vi "Agilent VNA Set Trigger Mode.vi"(6 "Channel":i8=1 min=1 max=99 step=1, 7 "Agilent VNA":T1, 8 "error in (no error)":errorcluster, 10 "Trigger Mode":T2, 11 "VISA Resource Name":refnum<visa-resource-name>) -> (0 "error out":errorcluster, 3 "dup VISA Resource Name":refnum<visa-resource-name>)   [LabVIEW 2011]
doc: "This VI for the HP8753B Network Analyzers reads the stimulus values. Except when performing log sweeps and freq list sweeps, this VI uses the start and stop values and the number of points to calcuate the stimulus values."
uses:
  TypeDefs/Agilent VNA Trigger Mode.ctl
  TypeDefs/Agilent VNA Instrument Info.ctl
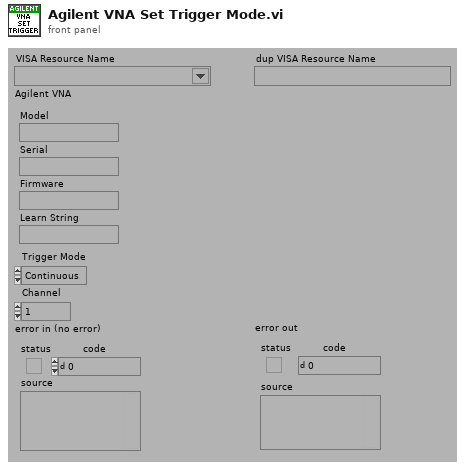
[diagram p1: front panel]
types:
  T1 = typedef "Agilent VNA Instrument Info.ctl" = cluster{"Model":string, "Serial":string, "Firmware":string, "Learn String":string}
  T2 = typedef "Agilent VNA Trigger Mode.ctl" = enum16{"Continuous", "Hold", "Single"}
  T3 = typedef "Agilent VNA Model.ctl" = enum16{"Not Supported", "8510X", "8719X", "8720X", "8722X", "8753X", "ENA", "PNA", "Field Fox"}
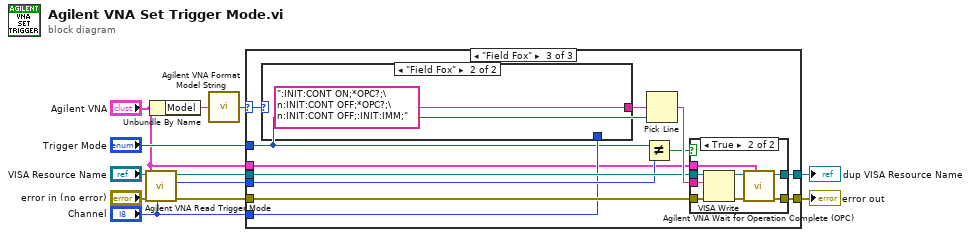
[diagram p0: block diagram]
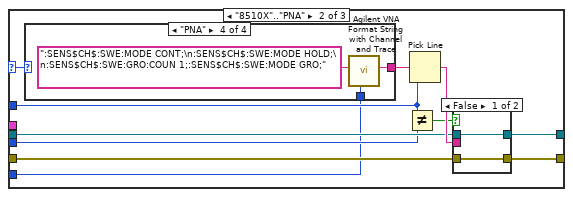
[diagram p3: hidden frame]
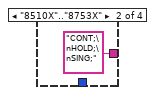
[diagram p5: hidden frame]
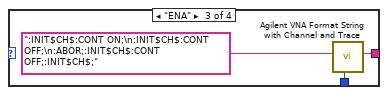
[diagram p6: hidden frame]
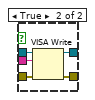
[diagram p7: hidden frame]
diagram:
  n1 = call "Agilent VNA Read Trigger Mode.vi"("Channel"="Channel", "Agilent VNA"="Agilent VNA", "error in (no error)"="error in (no error)", "VISA Resource Name"="VISA Resource Name") -> ("error out"=w7:errorcluster, "Trigger Mode"=w5:T2, "dup VISA Resource Name"=w6:refnum<visa-resource-name>)  [unwired: 5 out]
  n2 = Unbundle By Name("Agilent VNA") -> ("Model"=w3:string)
  n3 = call "Agilent VNA Format Model String.vi"("Model"=w3) -> ("Model"=w2:T3)
  n4 = case shown="\"Field Fox\"" w2 {
    selector: w2 -> [_ w15 w42]
    tunnel: [w13 w25 w51] -> w12
    tunnel: [w14 w24 w50] -> w11
    tunnel: "Trigger Mode" -> [_ w23 w40]
    tunnel: w7 -> [w14 w19 w46]
    tunnel: w6 -> [w13 w18 w45]
    tunnel: w5 -> [_ w17 w44]
    tunnel: "Channel" -> [_ w16 w43]
    tunnel: "Agilent VNA" -> [_ _ w41]
    frame "Not Supported" {
    }
    frame "8510X".."PNA" {
      n5 = case shown="\"PNA\"" w15 {
        tunnel: [_ "CONT;\nHOLD;\nSING;" w28 w31] -> w21
        tunnel: w16 -> [_ _ w27 w30]
        frame "Not Supported", "Field Fox" {
        }
        frame "8510X".."8753X" {
        }
        frame "ENA" {
          n6 = call "Agilent VNA Format String with Channel and Trace.vi"("Channel"=w27, "String"=":INIT$CH$:CONT ON;\n:INIT$CH$:CONT OFF;\n:ABOR;:INIT$CH$:CONT OFF;:INIT$CH$;") -> ("String Out"=w28:string)  [unwired: 1 in, 6 out]
        }
        frame "PNA" {
          n7 = call "Agilent VNA Format String with Channel and Trace.vi"("Channel"=w30, "String"=":SENS$CH$:SWE:MODE CONT;\n:SENS$CH$:SWE:MODE HOLD;\n:SENS$CH$:SWE:GRO:COUN 1;:SENS$CH$:SWE:MODE GRO;") -> ("String Out"=w31:string)  [unwired: 1 in, 6 out]
        }
      }
      n8 = Not Equal?(x=w23, y=w17) -> (x != y?=w20:bool)
      n9 = Pick Line(multi-line string=w21, line index=w23) -> (output string=w22:string)  [unwired: 1 out]
      n10 = case shown="False" w20 {
        tunnel: w19 -> [w33 w39]
        tunnel: w18 -> [w34 w38]
        tunnel: w22 -> [_ w37]
        tunnel: [w34 w36] -> w25
        tunnel: [w33 w35] -> w24
        frame False {
        }
        frame True {
          n11 = VISA Write(VISA resource name=w38, write buffer=w37, error in (no error)=w39) -> (VISA resource name out=w36:refnum<visa-resource-name>, error out=w35:errorcluster)  [unwired: 1 out]
        }
      }
    }
    frame "Field Fox" {
      n12 = case shown="\"Field Fox\"" w42 {
        tunnel: [_ ":INIT:CONT ON;*OPC?;\n:INIT:CONT OFF;*OPC?;\n:INIT:CONT OFF;:INIT:IMM;"] -> w48
        tunnel: w43 -> [_ _]
        frame "Not Supported".."PNA" {
        }
        frame "Field Fox" {
        }
      }
      n13 = Not Equal?(x=w40, y=w44) -> (x != y?=w47:bool)
      n14 = Pick Line(multi-line string=w48, line index=w40) -> (output string=w49:string)  [unwired: 1 out]
      n15 = case shown="True" w47 {
        tunnel: w46 -> [w53 w62]
        tunnel: w45 -> [w54 w61]
        tunnel: w49 -> [_ w60]
        tunnel: [w54 w57] -> w51
        tunnel: [w53 w56] -> w50
        tunnel: w41 -> [_ w55]
        frame False {
        }
        frame True {
          n16 = VISA Write(VISA resource name=w61, write buffer=w60, error in (no error)=w62) -> (VISA resource name out=w58:refnum<visa-resource-name>, error out=w59:errorcluster)  [unwired: 1 out]
          n17 = call "Agilent VNA Wait for Operation Complete (OPC).vi"("Agilent VNA"=w55, "error in (no error)"=w59, "VISA Resource Name"=w58) -> ("error out"=w56:errorcluster, "dup VISA Resource Name"=w57:refnum<visa-resource-name>)  [unwired: 1 in, 6 out]
        }
      }
    }
  }
  "dup VISA Resource Name" <- w12
  "error out" <- w11
